vi "Ej7.vi"() -> ()   [LabVIEW 2023]
panel:
  in  "stop":bool
  in  "Squarewave\nFrequency":dbl(slide) scale=0.0..1000.0
  in  "Sinewave \nFrequency":dbl(slide) scale=0.0..1000.0
  out "Waveform Graph":dynamicdata(graph)
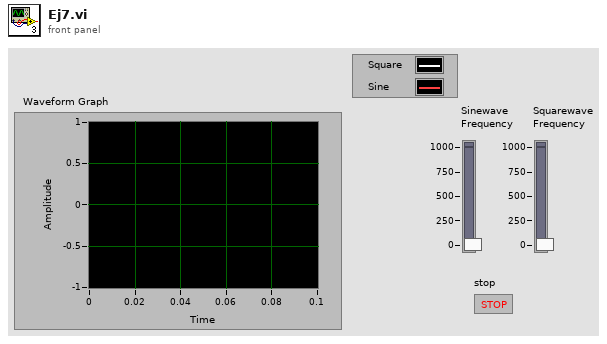
[diagram p1: front panel]
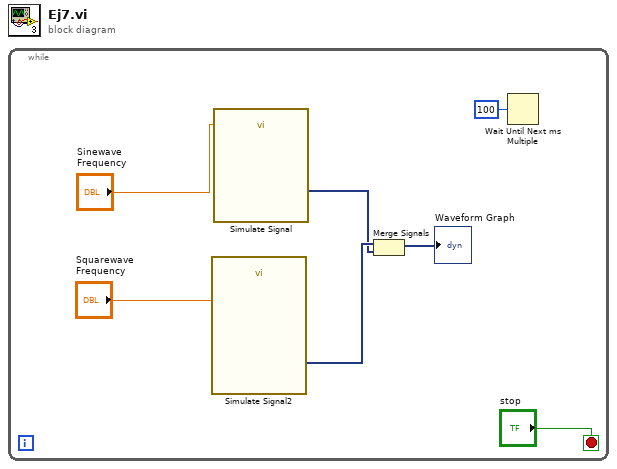
[diagram p0: block diagram]
diagram:
  n1 = while {
    stop <- "stop" stop-if-true
    n2 = call "Simulate Signal2"("Frequency"="Squarewave\nFrequency") -> ("Square"=w3:dynamicdata)  [unwired: 13 in, 1 out]
    n3 = call "Simulate Signal"("Frequency"="Sinewave \nFrequency") -> ("Sine"=w1:dynamicdata)  [unwired: 13 in, 1 out]
    n4 = Merge Signals(w3, w1) -> (→"Waveform Graph":dynamicdata)
    n5 = Wait Until Next ms Multiple(millisecond multiple=u32 100) -> ()  [unwired: 1 out]
  }
